vi "st_str Incorporate New Data.vi"(8 "error in (no error)":errorcluster, 9 "New Graph Data XY":cluster{"X":dbl[], "Y":dbl[]}[](array[cluster]), 10 "New Graph Data":waveform(dbl)[](array[waveform]), 11 "Data in":T1={"UI References"={"Exit Ref"=refnum, "Save Ref"=refnum, "Open Ref"=refnum, "Export Ref"=refnum, "Acquire Ref"=refnum, "Configure Ref"=refnum, "Graph Ref"=refnum, "Clear Ref"=refnum, "Analyze Ref"=refnum, "Status Ref"=refnum, "Snapshot Ref"=refnum, "Tbl Ref"=refnum, "XYGraph Ref"=refnum}, "Graph Data"={"Data"=[], "Annotation List"=[], "Cursor List"=[], "Analysis Data"=[], "XY graph"=[]}, "User Specified"={"Hardware Configuration"={"HW Refnum <Replace Me>"="", "Signal Type <Replace Me>"=enum."Sine Wave"}, "Analysis Configuration"={"Statistics"=TRUE}, "New Data Behavior"=enum."Replace"}, "GenParametr"={"UgenVrms"=0.0, "Frequency 1,kHz"=0.0, "dFreq, kHz"=0.0, "Frequency 2,kHz"=0.0, "WaitSignalGen"=0.0}}) -> (0 "error out":errorcluster, 3 "Data out":T1={"UI References"={"Exit Ref"=refnum, "Save Ref"=refnum, "Open Ref"=refnum, "Export Ref"=refnum, "Acquire Ref"=refnum, "Configure Ref"=refnum, "Graph Ref"=refnum, "Clear Ref"=refnum, "Analyze Ref"=refnum, "Status Ref"=refnum, "Snapshot Ref"=refnum, "Tbl Ref"=refnum, "XYGraph Ref"=refnum}, "Graph Data"={"Data"=[], "Annotation List"=[], "Cursor List"=[], "Analysis Data"=[], "XY graph"=[]}, "User Specified"={"Hardware Configuration"={"HW Refnum <Replace Me>"="", "Signal Type <Replace Me>"=enum."Sine Wave"}, "Analysis Configuration"={"Statistics"=TRUE}, "New Data Behavior"=enum."Replace"}, "GenParametr"={"UgenVrms"=0.0, "Frequency 1,kHz"=0.0, "dFreq, kHz"=0.0, "Frequency 2,kHz"=0.0, "WaitSignalGen"=0.0}})   [LabVIEW 2017]
doc: "Incorporates newly acquired or loaded data into the main state data. New data can replace, be appended to, or overlayed over (as an additional channel) existing data. If the user does not have a preference saved a dialog will be presented asking which method to use."
uses:
  controls/st_str Data.ctl
  controls/st_str UI References.ctl
  controls/st_str Graph Data.ctl
  <vilib>/Utility/miscctls.llb/LVAnnotationListTypeDef.ctl
  <vilib>/Utility/miscctls.llb/LVCursorListTypeDef.ctl
  controls/st_str User Specified Data.ctl
  controls/st_str HW Configuration.ctl
  controls/st_str Simulated Signal Type.ctl
  controls/st_str Analysis Configuration.ctl
  controls/st_str New Data Behavior.ctl
panel:
  # "(Scroll up to see large state data in/out clusters)"
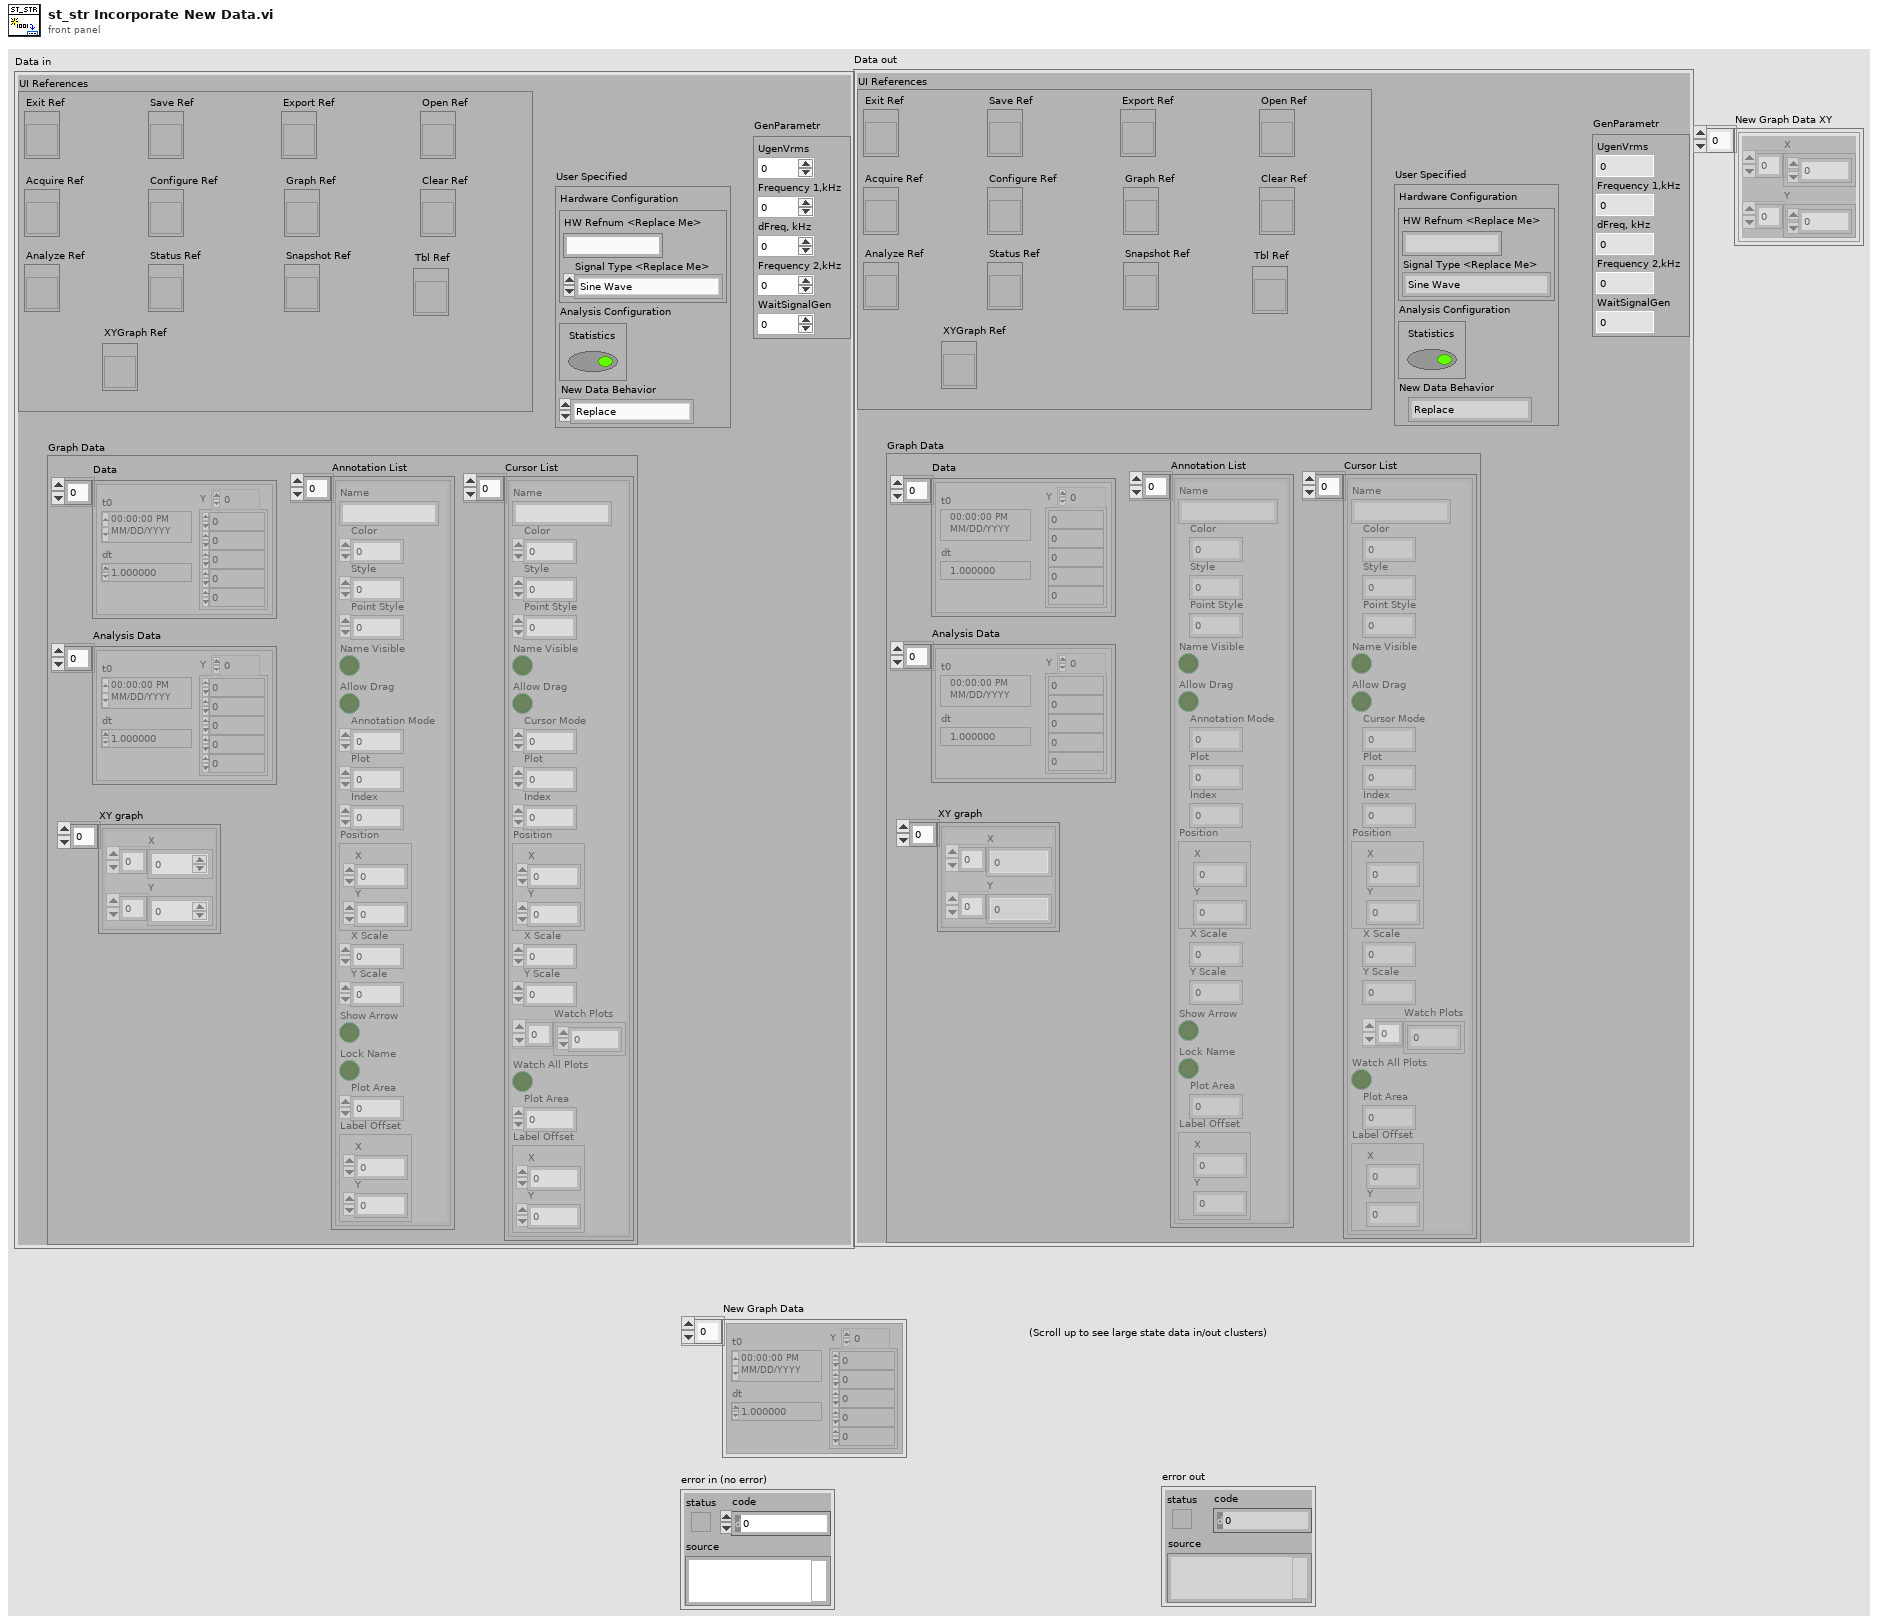
[diagram p1: front panel]
types:
  T1 = typedef "st_str Data.ctl" = cluster{"UI References":T2, "Graph Data":T3, "User Specified":T6, "GenParametr":cluster{"UgenVrms":dbl, "Frequency 1,kHz":dbl, "dFreq, kHz":dbl, "Frequency 2,kHz":dbl, "WaitSignalGen":dbl}}
  T2 = typedef "st_str UI References.ctl" = cluster{"Exit Ref":refnum<vi>, "Save Ref":refnum<vi>, "Open Ref":refnum<vi>, "Export Ref":refnum<vi>, "Acquire Ref":refnum<vi>, "Configure Ref":refnum<vi>, "Graph Ref":refnum<vi>, "Clear Ref":refnum<vi>, "Analyze Ref":refnum<vi>, "Status Ref":refnum<vi>, "Snapshot Ref":refnum<vi>, "Tbl Ref":refnum<vi>, "XYGraph Ref":refnum<vi>}
  T3 = typedef "st_str Graph Data.ctl" = cluster{"Data":waveform(dbl)[], "Annotation List":T4, "Cursor List":T5, "Analysis Data":waveform(dbl)[], "XY graph":cluster{"X":dbl[], "Y":dbl[]}[]}
  T4 = typedef "LVAnnotationListTypeDef.ctl" = cluster{"Name":string, "Color":u32, "Style":u8, "Point Style":u8, "Name Visible":bool, "Allow Drag":bool, "Annotation Mode":u32, "Plot":i32, "Index":i32, "Position":cluster{"X":dbl, "Y":dbl}, "X Scale":u32, "Y Scale":u32, "Show Arrow":bool, "Lock Name":bool, "Plot Area":i32, "Label Offset":cluster{"X":dbl, "Y":dbl}}[]
  T5 = typedef "LVCursorListTypeDef.ctl" = cluster{"Name":string, "Color":u32, "Style":u8, "Point Style":u8, "Name Visible":bool, "Allow Drag":bool, "Cursor Mode":u32, "Plot":i32, "Index":i32, "Position":cluster{"X":dbl, "Y":dbl}, "X Scale":u32, "Y Scale":u32, "Watch Plots":i32[], "Watch All Plots":bool, "Plot Area":i32, "Label Offset":cluster{"X":dbl, "Y":dbl}}[]
  T6 = typedef "st_str User Specified Data.ctl" = cluster{"Hardware Configuration":T7, "Analysis Configuration":T9, "New Data Behavior":T10}
  T7 = typedef "st_str HW Configuration.ctl" = cluster{"HW Refnum <Replace Me>":string, "Signal Type <Replace Me>":T8}
  T8 = typedef "st_str Simulated Signal Type.ctl" = enum16{"Sine Wave", "Square Wave"}
  T9 = typedef "st_str Analysis Configuration.ctl" = cluster{"Statistics":bool}
  T10 = typedef "st_str New Data Behavior.ctl" = enum16{"Replace", "Overlay", "Append"}
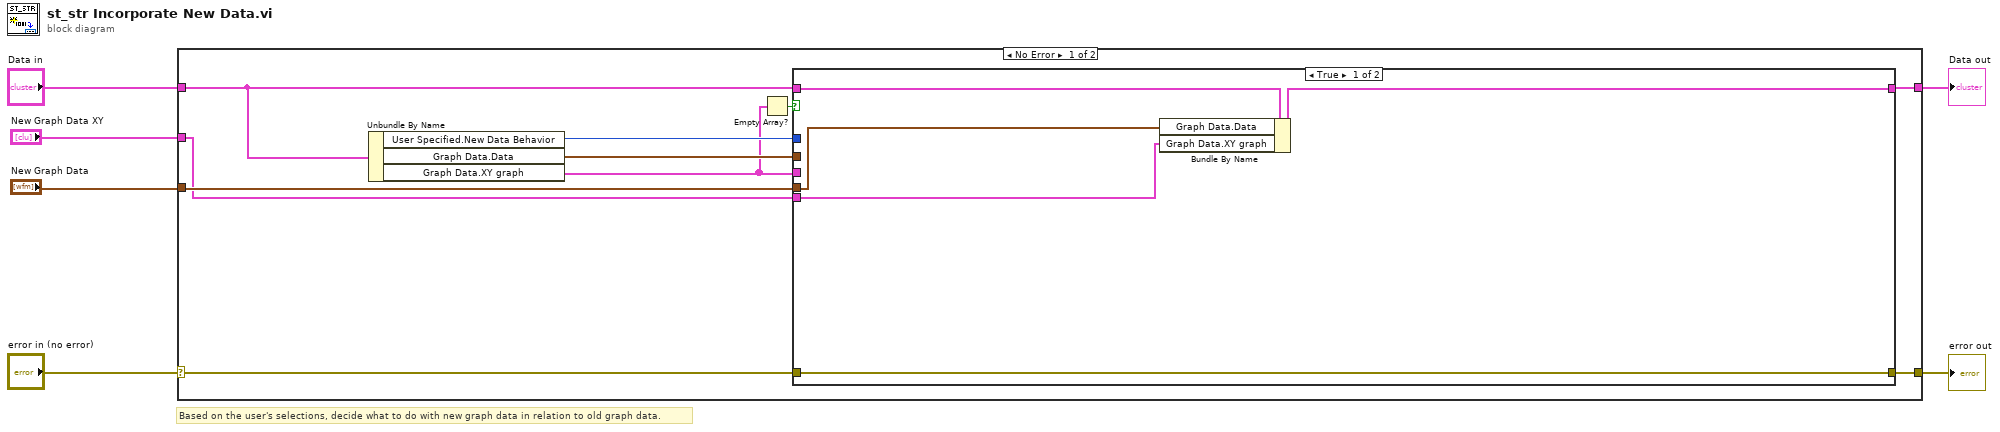
[diagram p0: block diagram]
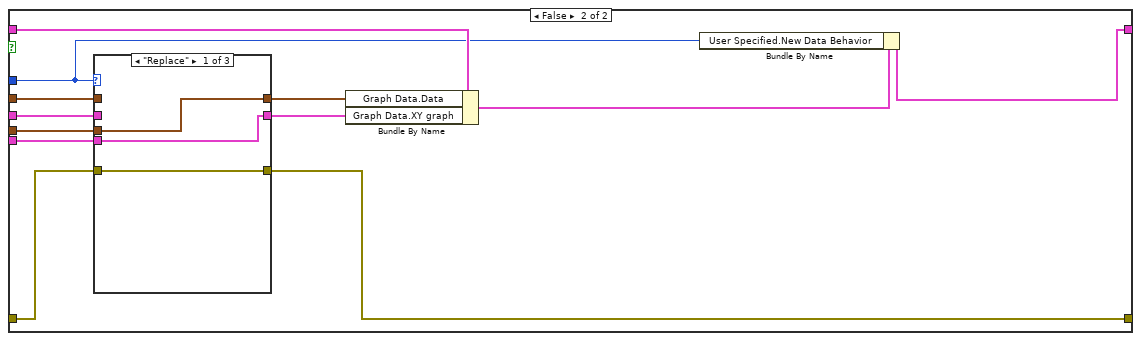
[diagram p2: hidden frame]
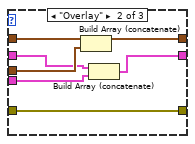
[diagram p3: hidden frame]
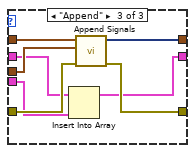
[diagram p4: hidden frame]
diagram:
  # "Based on the user's selections, decide what to do with new graph data in relation to old graph data."
  n1 = case shown="No Error" "error in (no error)" {
    selector: "error in (no error)" -> [w12 w53]
    tunnel: "Data in" -> [w16 w52]
    tunnel: "New Graph Data" -> [w14 _]
    tunnel: [w13 w52] -> w4
    tunnel: [w11 w53] -> w2
    tunnel: "New Graph Data XY" -> [w7 _]
    frame No Error {
      n2 = Unbundle By Name(w16) -> ("User Specified.New Data Behavior"=w15:T10, "Graph Data.Data"=w10:waveform(dbl)[], "Graph Data.XY graph"=w8:cluster{"X":dbl[], "Y":dbl[]}[])
      n3 = Empty Array?(array=w8) -> (empty?=w9:bool)
      n4 = case shown="True" w9 {
        tunnel: w16 -> [w21 w33]
        tunnel: w15 -> [_ w25]
        tunnel: w14 -> [w20 w32]
        tunnel: w10 -> [_ w30]
        tunnel: [w19 w28] -> w13
        tunnel: w12 -> [w18 w27]
        tunnel: [w18 w26] -> w11
        tunnel: w8 -> [_ w23]
        tunnel: w7 -> [w17 w22]
        frame True {
          n5 = Bundle By Name(cluster=w21, "Graph Data.Data"=w20, "Graph Data.XY graph"=w17) -> (w19:T1)
        }
        frame False {
          n6 = case shown="\"Replace\"" w25 {
            tunnel: w32 -> [w36 w42 w50]
            tunnel: [w36 w41 w49] -> w31
            tunnel: w30 -> [_ w43 w51]
            tunnel: w27 -> [w35 w40 w48]
            tunnel: [w35 w40 w47] -> w26
            tunnel: [w34 w37 w44] -> w24
            tunnel: w23 -> [_ w39 w46]
            tunnel: w22 -> [w34 w38 w45]
            frame "Replace" {
            }
            frame "Overlay" {
              n7 = Build Array (concatenate)(w43, w42) -> (w41:waveform(dbl)[])
              n8 = Build Array (concatenate)(w39, w38) -> (w37:cluster{"X":dbl[], "Y":dbl[]}[])
            }
            frame "Append" {
              n9 = Insert Into Array(array=w46, new element=w45) -> (w44:cluster{"X":dbl[], "Y":dbl[]}[])  [unwired: 1 in]
              n10 = call "Append Signals"("error in (no error)"=w48, "Input Signal B"=w50, "Input Signal A"=w51) -> ("error out"=w47:errorcluster, "Appended Signals"=w49:dynamicdata)  [unwired: 7 in]
            }
          }
          n11 = Bundle By Name(cluster=w33, "Graph Data.Data"=w31, "Graph Data.XY graph"=w24) -> (w29:T1)
          n12 = Bundle By Name(cluster=w29, "User Specified.New Data Behavior"=w25) -> (w28:T1)
        }
      }
    }
    frame Error {
    }
  }
  "Data out" <- w4
  "error out" <- w2
